vi "CalculateCurves.vi"(0 "Graph Sel":u16(ring) items=["Insertion Loss", "Group Delay", "Chromatic Dispersion", "Polarization Dependent Loss", "Polarization Mode Dispersion", "Linear Phase Deviation", "Quadratic Phase Deviation", "Jones Matrix Element Amplitudes", "Jones Matrix Element Phases", "Time Domain Amplitude", "Time Domain Wavelength", "Min/Max Loss", "Second Order PMD", "Phase Ripple Linear", "Phase Ripple Quadratic"], 1 "X-axis units":T1, 2 "Group Index":dbl=1.5 format="%.2f", 3 "res BW (GHz)":dbl format="%.2f", 4 "filter?":bool) -> (5 "Graph Data":cluster{dbl[], dbl[]}[](array[cluster]) {"?" format="%.2f"; "?" format="%.2f"}, 6 "genOutput":dbl[](array[numeric]) format="%.2f")   [LabVIEW 2024]
uses:
  X-Scales.ctl
  Program Files (x86)/Luna Technologies/OVA 5000 v5.14.2/data/OVA32.dll
panel:
  in  "genInput":dbl[](array[numeric])=[0.0, 0.0, 0.0, 0.0, 0.0, 0.0, 0.0, 0.0, 0.0, 0.0] format="%.2f"
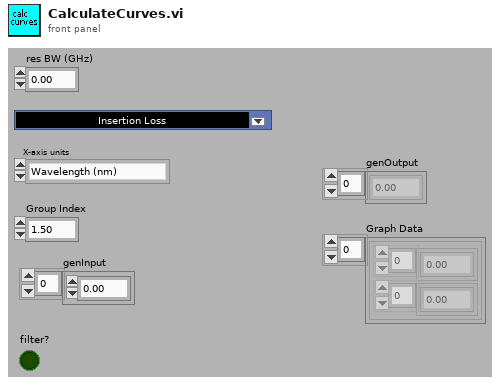
[diagram p1: front panel]
types:
  T1 = typedef "X-Scales.ctl" = enum16{"Wavelength (nm)", "Gigahertz (GHz)", "Terahertz (THz)", "Time (ns)", "Length (m)"}
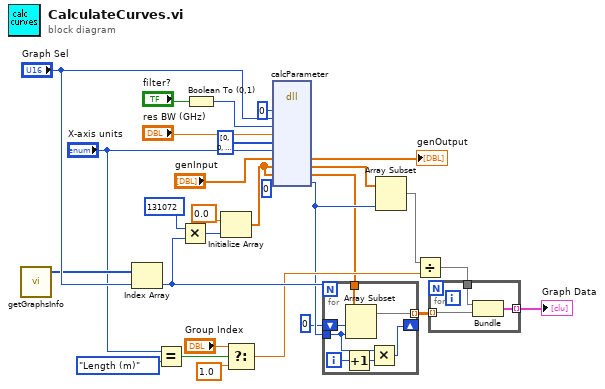
[diagram p0: block diagram]
diagram:
  n1 = call "getGraphsInfo.vi"() -> ("noOFCurvesInEachGraph"=w27:u32[])  [unwired: 1 in, 2 out]
  n2 = Index Array(array=w27, index="Graph Sel") -> (element=w26:u32)
  n3 = Equal?(x="X-axis units", y=X-Scales."Length (m)" ("X-axis scale")) -> (x = y?=w24:bool)
  n4 = Multiply(x=u32 131072 ("y"), y=w26) -> (x*y=w16:u32)
  n5 = Boolean To (0,1)(Boolean="filter?") -> (0, 1=w1:i16)
  n6 = Initialize Array(0.0 ("Element Data"), w16) -> (w19:dbl[])
  n7 = Select(t="Group Index", s=w24, f=1.0) -> (s? t:f=w25:dbl)
  n8 = dll-call lib="C:/Program Files (x86)/Luna Technologies/OVA 5000 v5.14.2/data/OVA32.dll" fn="calcParameter"("matrix"=u8 0, "graphs (params)"="Graph Sel", "filter"=w1, "res BW (GHz)"="res BW (GHz)", "indices"=u32[] [0, 0, 0, 0], "xAxisUnits"="X-axis units", "genOutput"="genInput", "xData"=w19, "yData"=w19, "segSize"=u32 0) -> ("genOutput"=→"genOutput":dbl[], "xData"=w11:dbl[], "yData"=w3:dbl[], "segSize"=w9:u32)  [unwired: 10 in, 2 out]
  n9 = for {
    N: w26 -> [_]
    tunnel: [w35] -> w5 mode=indexing
    tunnel: w3 -> [w36]
    shift-right: [w32] -> _
    shift-left: 0 -> [w30]
    tunnel: w9 -> [w33]
    i -> [w34]
    n10 = Increment(x=w34) -> (x+1=w31:i32)
    n11 = Array Subset(array=w36, index=w30, length=w33) -> (w35:dbl[])
    n12 = Multiply(x=w33, y=w31) -> (x*y=w32:u32)
  }
  n13 = Array Subset(array=w11, length=w9) -> (w10:dbl[])  [unwired: 1 in]
  n14 = Divide(x=w10, y=w25) -> (x/y=w7:dbl[])
  n15 = for {
    tunnel: w5 -> [w38] mode=indexing
    tunnel: w7 -> [w39]
    tunnel: [w37] -> w29 mode=indexing
    n16 = Bundle(w39, w38) -> (w37:cluster{dbl[], dbl[]})  [unwired: 1 in]
  }
  "Graph Data" <- w29
